vi "Check Network Connection.vi"(9 "CD Path":string, 10 "IP Address":string, 11 "Comm.Info":T1) -> (0 "error out":errorcluster, 3 "Comm.Info":T1)   [LabVIEW 2019, in "Instrument Workspace Shared.lvlib"]
uses:
  Instrument Workspace Shared.lvlib
  <vilib>/NI/STM/TCP/TCP Connection Info.ctl
  <vilib>/NI/STM/SubVIs/MetaDataElement.ctl
  APIs/Host Automation API/Instrument Host Automation API.lvlib
  <vilib>/NI/STM/NI STM.lvlib
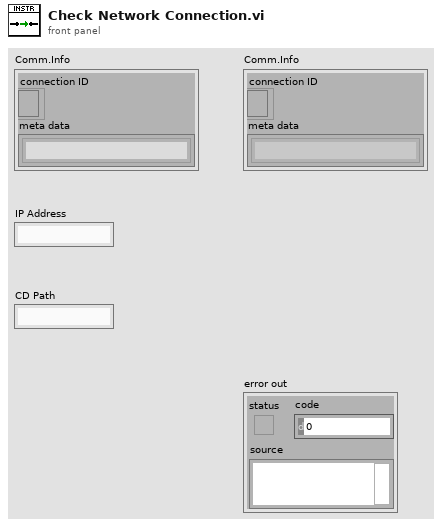
[diagram p1: front panel]
types:
  T1 = typedef "NI STM.lvlib/TCP Connection Info.ctl" = cluster{"connection ID":refnum<k5>, "meta data":T2[]}
  T2 = typedef "NI STM.lvlib/MetaDataElement.ctl" = string
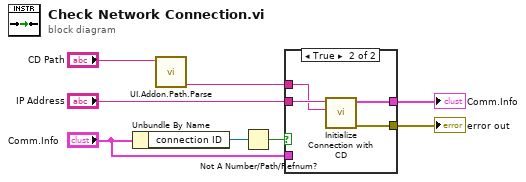
[diagram p0: block diagram]
diagram:
  n1 = Unbundle By Name("Comm.Info") -> ("connection ID"=w3:refnum<k5>)
  n2 = call "UI.Addon.Path.Parse.vi"("Cached Addon Path"="CD Path") -> ("Addon Name"=w1:string)  [unwired: 6 in, 4 out]
  n3 = Not A Number/Path/Refnum?(number/path/refnum=w3) -> (NaN/Path/Refnum?=w7:bool)
  n4 = case shown="True" w7 {
    tunnel: w1 -> [_ w12]
    tunnel: [w9 w10] -> w5
    tunnel: "Comm.Info" -> [w9 _]
    tunnel: [_ w11] -> w8
    tunnel: "IP Address" -> [_ w13]
    frame False {
    }
    frame True {
      n5 = call "Initialize Connection with CD.vi"("TCP Service"=w12, "IP Address"=w13) -> ("error out"=w11:errorcluster, "connection info out"=w10:T1)  [unwired: 8 in]
    }
  }
  "error out" <- w8
  "Comm.Info" <- w5
